vi "HW_GEN - Generate Device info from File and Hardware.vi"(10 "QXdevInfo":T1, 11 "FileDevInfo[]":T1[](array[typedef])) -> (3 "DevInfo[] out":T1[](array[typedef]))   [LabVIEW 2016]
uses:
  Ctrls/HardWare Basic Info _ Channel.ctl
  Ctrls/HardWare Basic Info _ Module.ctl
  Ctrls/HardWare Basic Info _ Chassis.ctl
  Ctrls/HardWare Basic Info _ Device.ctl
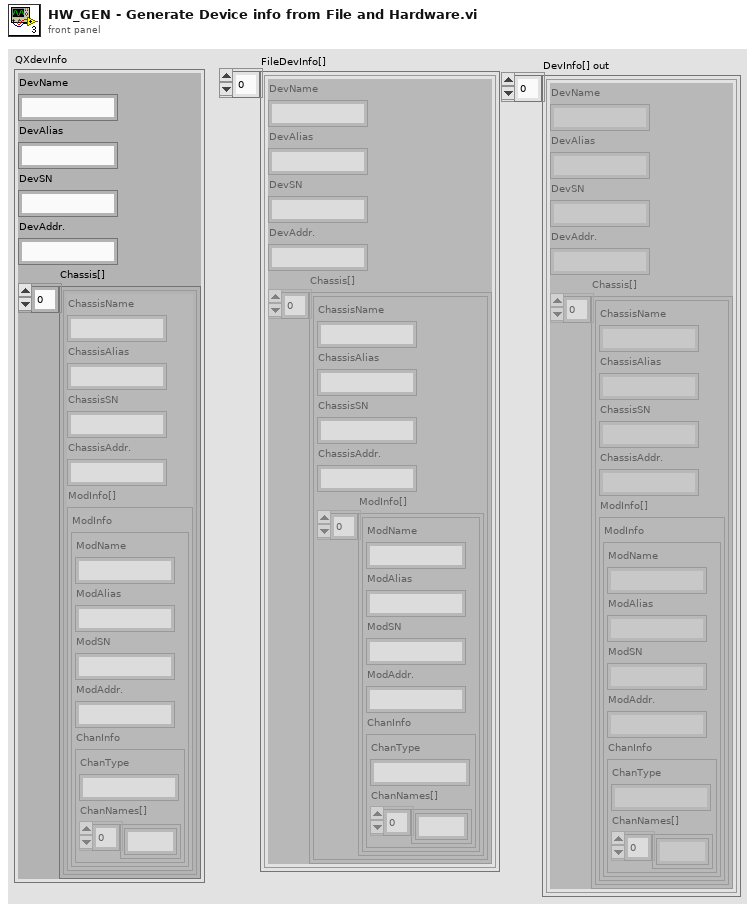
[diagram p1: front panel]
types:
  T1 = typedef "HardWare Basic Info _ Device.ctl" = cluster{"DevName":string, "DevAlias":string, "DevSN":string, "DevAddr.":string, "Chassis[]":T2[]}
  T2 = typedef "HardWare Basic Info _ Chassis.ctl" = cluster{"ChassisName":string, "ChassisAlias":string, "ChassisSN":string, "ChassisAddr.":string, "ModInfo[]":T3[]}
  T3 = typedef "HardWare Basic Info _ Module.ctl" = cluster{"ModName":string, "ModAlias":string, "ModSN":string, "ModAddr.":string, "ChanInfo":T4}
  T4 = typedef "HardWare Basic Info _ Channel.ctl" = cluster{"ChanType":string, "ChanNames[]":string[]}
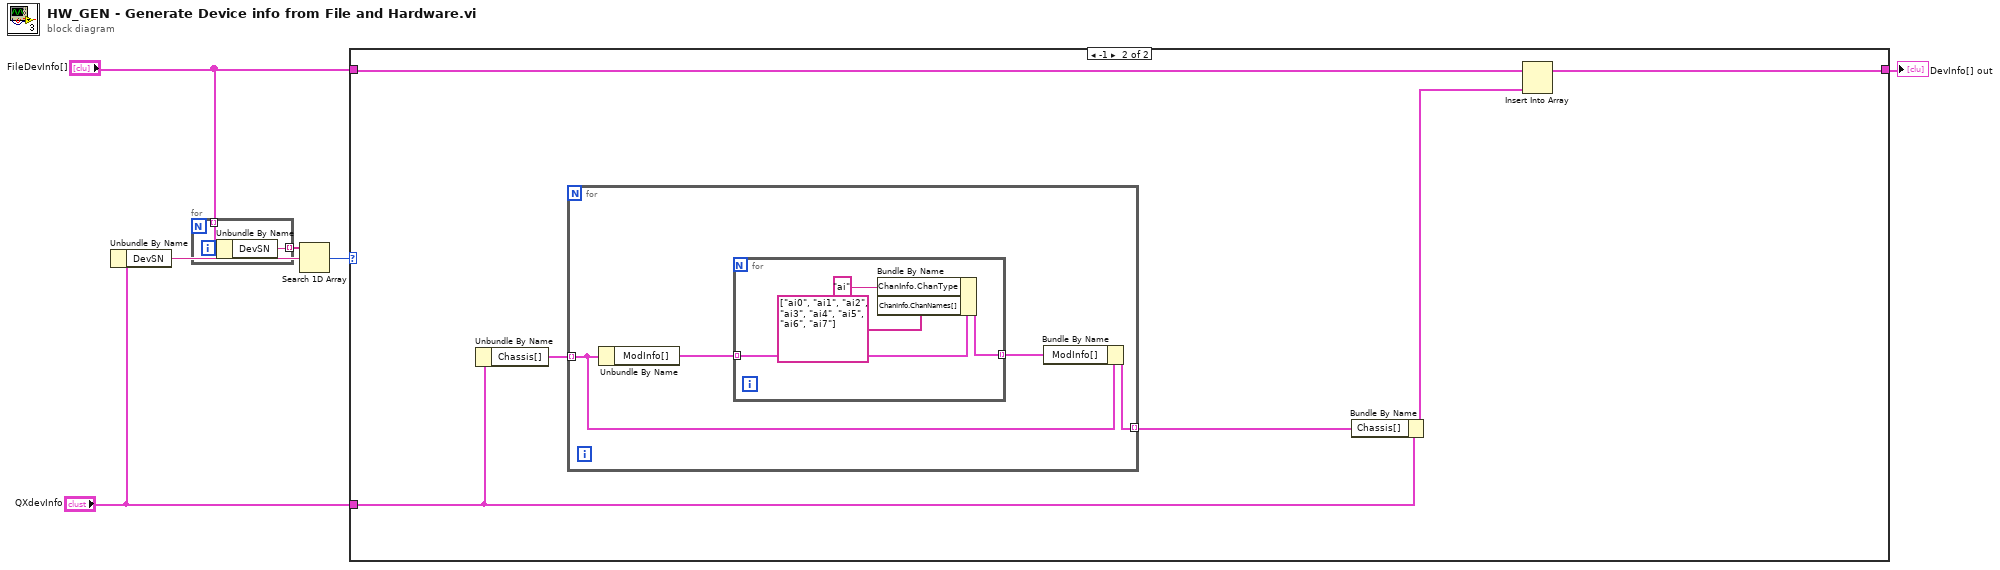
[diagram p0: block diagram]
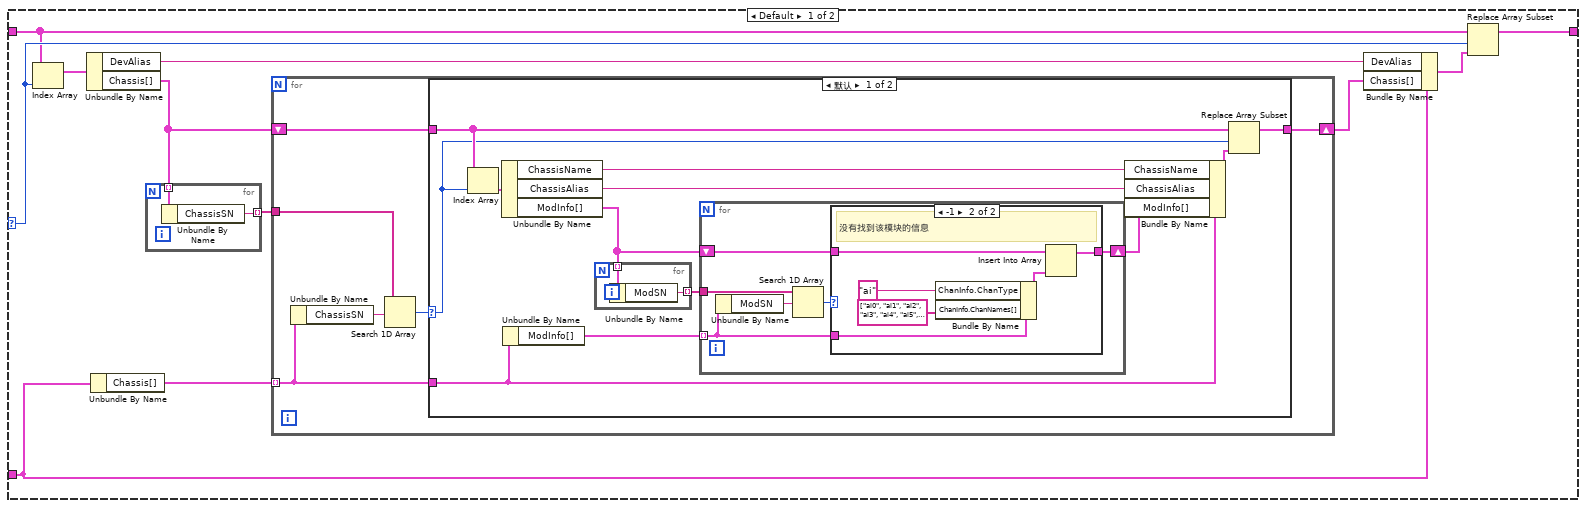
[diagram p2: hidden frame]
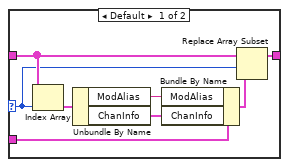
[diagram p3: hidden frame]
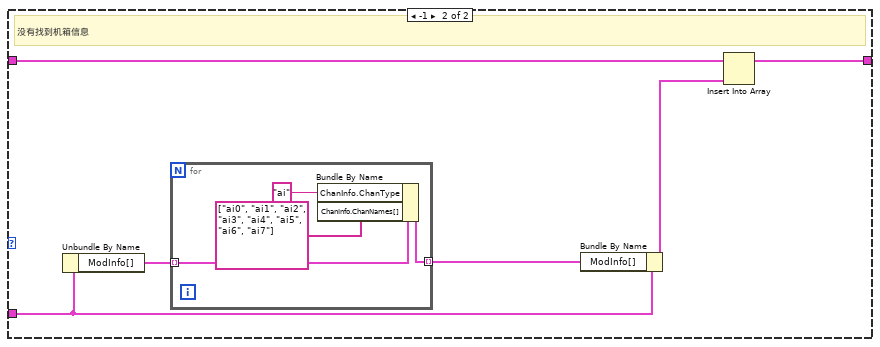
[diagram p4: hidden frame]
diagram:
  n1 = Unbundle By Name("QXdevInfo") -> ("DevSN"=w4:string)
  n2 = for {
    tunnel: "FileDevInfo[]" -> [w8] mode=indexing
    tunnel: [w7] -> w5 mode=indexing
    n3 = Unbundle By Name(w8) -> ("DevSN"=w7:string)
  }
  n4 = Search 1D Array(1D array=w5, element=w4) -> (index of element=w3:i32)  [unwired: 1 in]
  n5 = case shown="-1" w3 {
    selector: w3 -> [w13 _]
    tunnel: "QXdevInfo" -> [w11 w76]
    tunnel: "FileDevInfo[]" -> [w12 w74]
    tunnel: [w9 w72] -> w1
    frame Default {
      n6 = Index Array(array=w12, index=w13) -> (element=w15:T1)
      n7 = Unbundle By Name(w15) -> ("DevAlias"=w19:string, "Chassis[]"=w16:T2[])
      n8 = Unbundle By Name(w11) -> ("Chassis[]"=w17:T2[])
      n9 = for {
        tunnel: w16 -> [w71] mode=indexing
        tunnel: [w70] -> w18 mode=indexing
        n10 = Unbundle By Name(w71) -> ("ChassisSN"=w70:string)
      }
      n11 = for {
        tunnel: w18 -> [w25]
        tunnel: w17 -> [w21] mode=indexing
        shift-right: [w20] -> w14
        shift-left: w16 -> [w22]
        n12 = Unbundle By Name(w21) -> ("ChassisSN"=w24:string)
        n13 = Search 1D Array(1D array=w25, element=w24) -> (index of element=w23:i32)  [unwired: 1 in]
        n14 = case shown="默认" w23 {
          selector: w23 -> [w28 _]
          tunnel: w22 -> [w30 w62]
          tunnel: w21 -> [w34 w65]
          tunnel: [w29 w61] -> w20
          frame Default {
            n15 = Index Array(array=w30, index=w28) -> (element=w37:T2)
            n16 = Unbundle By Name(w37) -> ("ChassisName"=w36:string, "ChassisAlias"=w35:string, "ModInfo[]"=w31:T3[])
            n17 = Unbundle By Name(w34) -> ("ModInfo[]"=w32:T3[])
            n18 = for {
              tunnel: w31 -> [w59] mode=indexing
              tunnel: [w58] -> w33 mode=indexing
              n19 = Unbundle By Name(w59) -> ("ModSN"=w58:string)
            }
            n20 = for {
              tunnel: w33 -> [w43]
              tunnel: w32 -> [w39] mode=indexing
              shift-right: [w38] -> w26
              shift-left: w31 -> [w40]
              n21 = Unbundle By Name(w39) -> ("ModSN"=w42:string)
              n22 = Search 1D Array(1D array=w43, element=w42) -> (index of element=w41:i32)  [unwired: 1 in]
              n23 = case shown="-1" w41 {
                selector: w41 -> [w44 _]
                tunnel: w40 -> [w47 w53]
                tunnel: w39 -> [w50 w57]
                tunnel: [w46 w54] -> w38
                frame Default {
                  n24 = Index Array(array=w47, index=w44) -> (element=w51:T3)
                  n25 = Unbundle By Name(w51) -> ("ModAlias"=w48:string, "ChanInfo"=w49:T4)
                  n26 = Bundle By Name(cluster=w50, "ModAlias"=w48, "ChanInfo"=w49) -> (w45:T3)
                  n27 = Replace Array Subset(array=w47, new element=w45, index=w44) -> (w46:T3[])
                }
                frame -1 {
                  # "没有找到该模块的信息"
                  n28 = Bundle By Name(cluster=w57, "ChanInfo.ChanType"="ai", "ChanInfo.ChanNames[]"=string[] ["ai0", "ai1", "ai2", "ai3", "ai4", "ai5", "ai6", "ai7"]) -> (w52:T3)
                  n29 = Insert Into Array(array=w53, new element=w52) -> (w54:T3[])  [unwired: 1 in]
                }
              }
            }
            n30 = Bundle By Name(cluster=w34, "ChassisName"=w36, "ChassisAlias"=w35, "ModInfo[]"=w26) -> (w27:T2)
            n31 = Replace Array Subset(array=w30, new element=w27, index=w28) -> (w29:T2[])
          }
          frame -1 {
            # "没有找到机箱信息"
            n32 = Unbundle By Name(w65) -> ("ModInfo[]"=w64:T3[])
            n33 = for {
              tunnel: w64 -> [w67] mode=indexing
              tunnel: [w66] -> w63 mode=indexing
              n34 = Bundle By Name(cluster=w67, "ChanInfo.ChanType"="ai", "ChanInfo.ChanNames[]"=string[] ["ai0", "ai1", "ai2", "ai3", "ai4", "ai5", "ai6", "ai7"]) -> (w66:T3)
            }
            n35 = Bundle By Name(cluster=w65, "ModInfo[]"=w63) -> (w60:T2)
            n36 = Insert Into Array(array=w62, new element=w60) -> (w61:T2[])  [unwired: 1 in]
          }
        }
      }
      n37 = Bundle By Name(cluster=w11, "DevAlias"=w19, "Chassis[]"=w14) -> (w10:T1)
      n38 = Replace Array Subset(array=w12, new element=w10, index=w13) -> (w9:T1[])
    }
    frame -1 {
      n39 = Unbundle By Name(w76) -> ("Chassis[]"=w77:T2[])
      n40 = for {
        tunnel: w77 -> [w79] mode=indexing
        tunnel: [w80] -> w75 mode=indexing
        n41 = Unbundle By Name(w79) -> ("ModInfo[]"=w81:T3[])
        n42 = for {
          tunnel: w81 -> [w83] mode=indexing
          tunnel: [w82] -> w78 mode=indexing
          n43 = Bundle By Name(cluster=w83, "ChanInfo.ChanType"="ai", "ChanInfo.ChanNames[]"=string[] ["ai0", "ai1", "ai2", "ai3", "ai4", "ai5", "ai6", "ai7"]) -> (w82:T3)
        }
        n44 = Bundle By Name(cluster=w79, "ModInfo[]"=w78) -> (w80:T2)
      }
      n45 = Bundle By Name(cluster=w76, "Chassis[]"=w75) -> (w73:T1)
      n46 = Insert Into Array(array=w74, new element=w73) -> (w72:T1[])  [unwired: 1 in]
    }
  }
  "DevInfo[] out" <- w1
